vi "T564_On-OffFromQueryResponseString.vi"(11 "String":string) -> (3 "ChannelON?":bool)   [LabVIEW 2013]
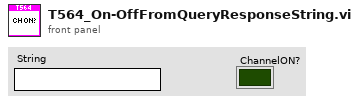
[diagram p1: front panel]
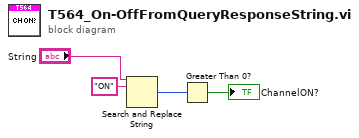
[diagram p0: block diagram]
diagram:
  n1 = Search and Replace String(input string="String", search string="ON") -> (number of replacements=w2:i32)  [unwired: 6 in, 3 out]
  n2 = Greater Than 0?(x=w2) -> (x > 0?=→"ChannelON?":bool)
